vi "Parameters.vi"() -> ()   [LabVIEW 2018]
uses:
  Class 2.lvclass
panel:
  out "A/Z":dbl
  out "A/Z 3":dbl
  in  "Z2 6":dbl=3.0
  in  "A2 6":dbl=16.0
  out "Im 8":dbl format="%#.3f"
  out "B0(T) 8":dbl format="%#.3f"
  out "B0(kGs) 8":dbl format="%#.3f"
  out "MeV/u 8":dbl format="%#.3f"
  out "F 8":dbl format="%#.3f"
  out "A/Z 8":dbl format="%#.3f"
  out "E (MeV)2 6":dbl format="%#.3f"
  out "Udef 8":dbl format="%#.3f"
  out "Uinfl 8":dbl format="%#.3f"
  out "Ubender 8":dbl format="%#.3f"
  out "UIAT 8":dbl format="%#.3f"
  out "Uinj 8":dbl format="%#.3f"
  in  "Z2 5":dbl=2.0
  in  "A2 5":dbl=12.0
  out "Im 7":dbl format="%#.3f"
  out "B0(T) 7":dbl format="%#.3f"
  out "B0(kGs) 7":dbl format="%#.3f"
  out "MeV/u 7":dbl format="%#.3f"
  out "F 7":dbl format="%#.3f"
  out "A/Z 7":dbl format="%#.3f"
  out "E (MeV)2 5":dbl format="%#.3f"
  out "Udef 7":dbl format="%#.3f"
  out "Uinfl 7":dbl format="%#.3f"
  out "Ubender 7":dbl format="%#.3f"
  out "UIAT 7":dbl format="%#.3f"
  out "Uinj 7":dbl format="%#.3f"
  in  "Z":dbl=3.0
  in  "A":dbl=14.0
  out "Im 6":dbl format="%#.3f"
  out "B0(T) 6":dbl format="%#.3f"
  out "B0(kGs) 6":dbl format="%#.3f"
  out "MeV/u 6":dbl format="%#.3f"
  out "F 6":dbl format="%#.3f"
  out "A/Z 6":dbl format="%#.3f"
  out "E (MeV)2 4":dbl format="%#.3f"
  out "Udef 6":dbl format="%#.3f"
  out "Uinfl 6":dbl format="%#.3f"
  out "Ubender 6":dbl format="%#.3f"
  out "UIAT 6":dbl format="%#.3f"
  out "Uinj 6":dbl format="%#.3f"
  in  "Z2 3":dbl=3.0
  in  "A2 3":dbl=16.0
  out "Im 5":dbl format="%#.3f"
  out "B0(T) 5":dbl format="%#.3f"
  out "B0(kGs) 5":dbl format="%.3f"
  out "MeV/u 5":dbl format="%#.3f"
  out "F 5":dbl format="%#.3f"
  out "A/Z 5":dbl format="%#.3f"
  out "E (MeV)2 3":dbl format="%#.3f"
  out "Udef 5":dbl format="%#.3f"
  out "Uinfl 5":dbl format="%#.3f"
  out "Ubender 5":dbl format="%#.3f"
  out "UIAT 5":dbl format="%#.3f"
  out "Uinj 5":dbl format="%#.3f"
  out "E (MeV)2 2":dbl format="%#.3f"
  in  "Z2 2":dbl=2.0
  in  "A2 2":dbl=12.0
  out "Udef 4":dbl format="%#.3f"
  out "Uinfl 4":dbl format="%#.3f"
  out "Ubender 4":dbl format="%#.3f"
  out "UIAT 4":dbl format="%#.3f"
  out "Uinj 4":dbl format="%#.3f"
  out "Im 4":dbl format="%#.3f"
  out "B0(T) 4":dbl format="%#.3f"
  out "B0(kGs) 4":dbl format="%.3f"
  out "MeV/u 4":dbl format="%#.3f"
  out "F 4":dbl format="%#.3f"
  out "A/Z 4":dbl format="%#.3f"
  out "E (MeV)2":dbl format="%#.3f"
  in  "Z":dbl=3.0
  in  "A":dbl=14.0
  out "Udef 3":dbl format="%#.3f"
  out "Uinfl 3":dbl format="%#.3f"
  out "Ubender 3":dbl format="%#.3f"
  out "UIAT 3":dbl format="%#.3f"
  out "Uinj 3":dbl format="%#.3f"
  out "Im 3":dbl format="%#.3f"
  out "B0(T) 3":dbl format="%#.3f"
  out "B0(kGs) 3":dbl format="%.3f"
  out "MeV/u 3":dbl format="%#.3f"
  out "F 3":dbl format="%#.3f"
  in  "Rm":dbl=9.2
  out "Udef":dbl format="%#.3f"
  out "Uinfl":dbl format="%#.3f"
  out "Ubender":dbl format="%#.3f"
  out "UIAT":dbl format="%#.3f"
  out "Uinj":dbl format="%#.3f"
  out "Im":dbl format="%#.3f"
  out "B0(T)":dbl format="%#.3f"
  out "B0(kGs)":dbl format="%#.3f"
  out "MeV/u":dbl format="%#.3f"
  out "F":dbl format="%#.3f"
  out "A/Z":dbl format="%#.3f"
  in  "Rm":dbl=7.5
  out "Udef":dbl format="%#.3f"
  out "Uinfl":dbl format="%#.3f"
  out "Ubender":dbl format="%#.3f"
  out "UIAT":dbl format="%#.3f"
  out "Uinj":dbl format="%#.3f"
  out "Im":dbl format="%#.3f"
  out "B0(T)":dbl format="%#.3f"
  out "B0(kGs)":dbl format="%.3f"
  out "MeV/u":dbl format="%#.3f"
  out "F":dbl format="%#.3f"
  in  "stop":bool
  in  "HARM":dbl=3.0
  in  "UECR":dbl=15.0
  in  "E (MeV)":dbl=255.0
  in  "Rextr":dbl=1.78
  in  "Z":dbl=10.0
  in  "A":dbl=48.0
  # "Инфлектор типа A"
  # "Инфлектор типа B"
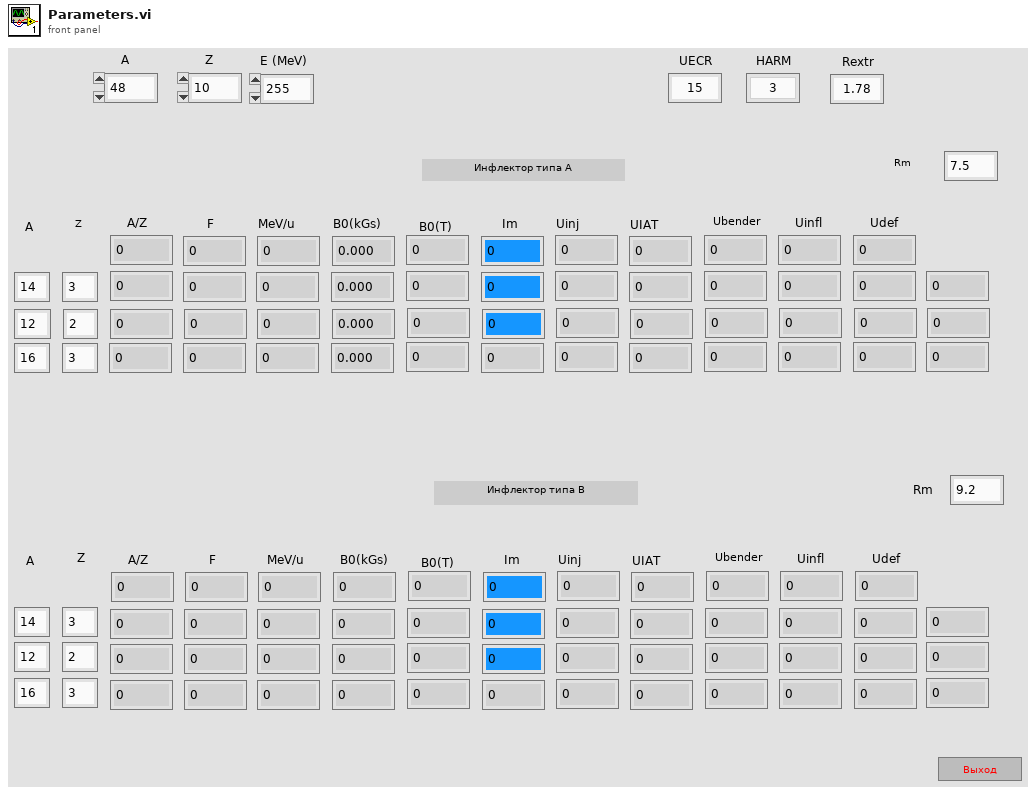
[diagram p1: front panel]
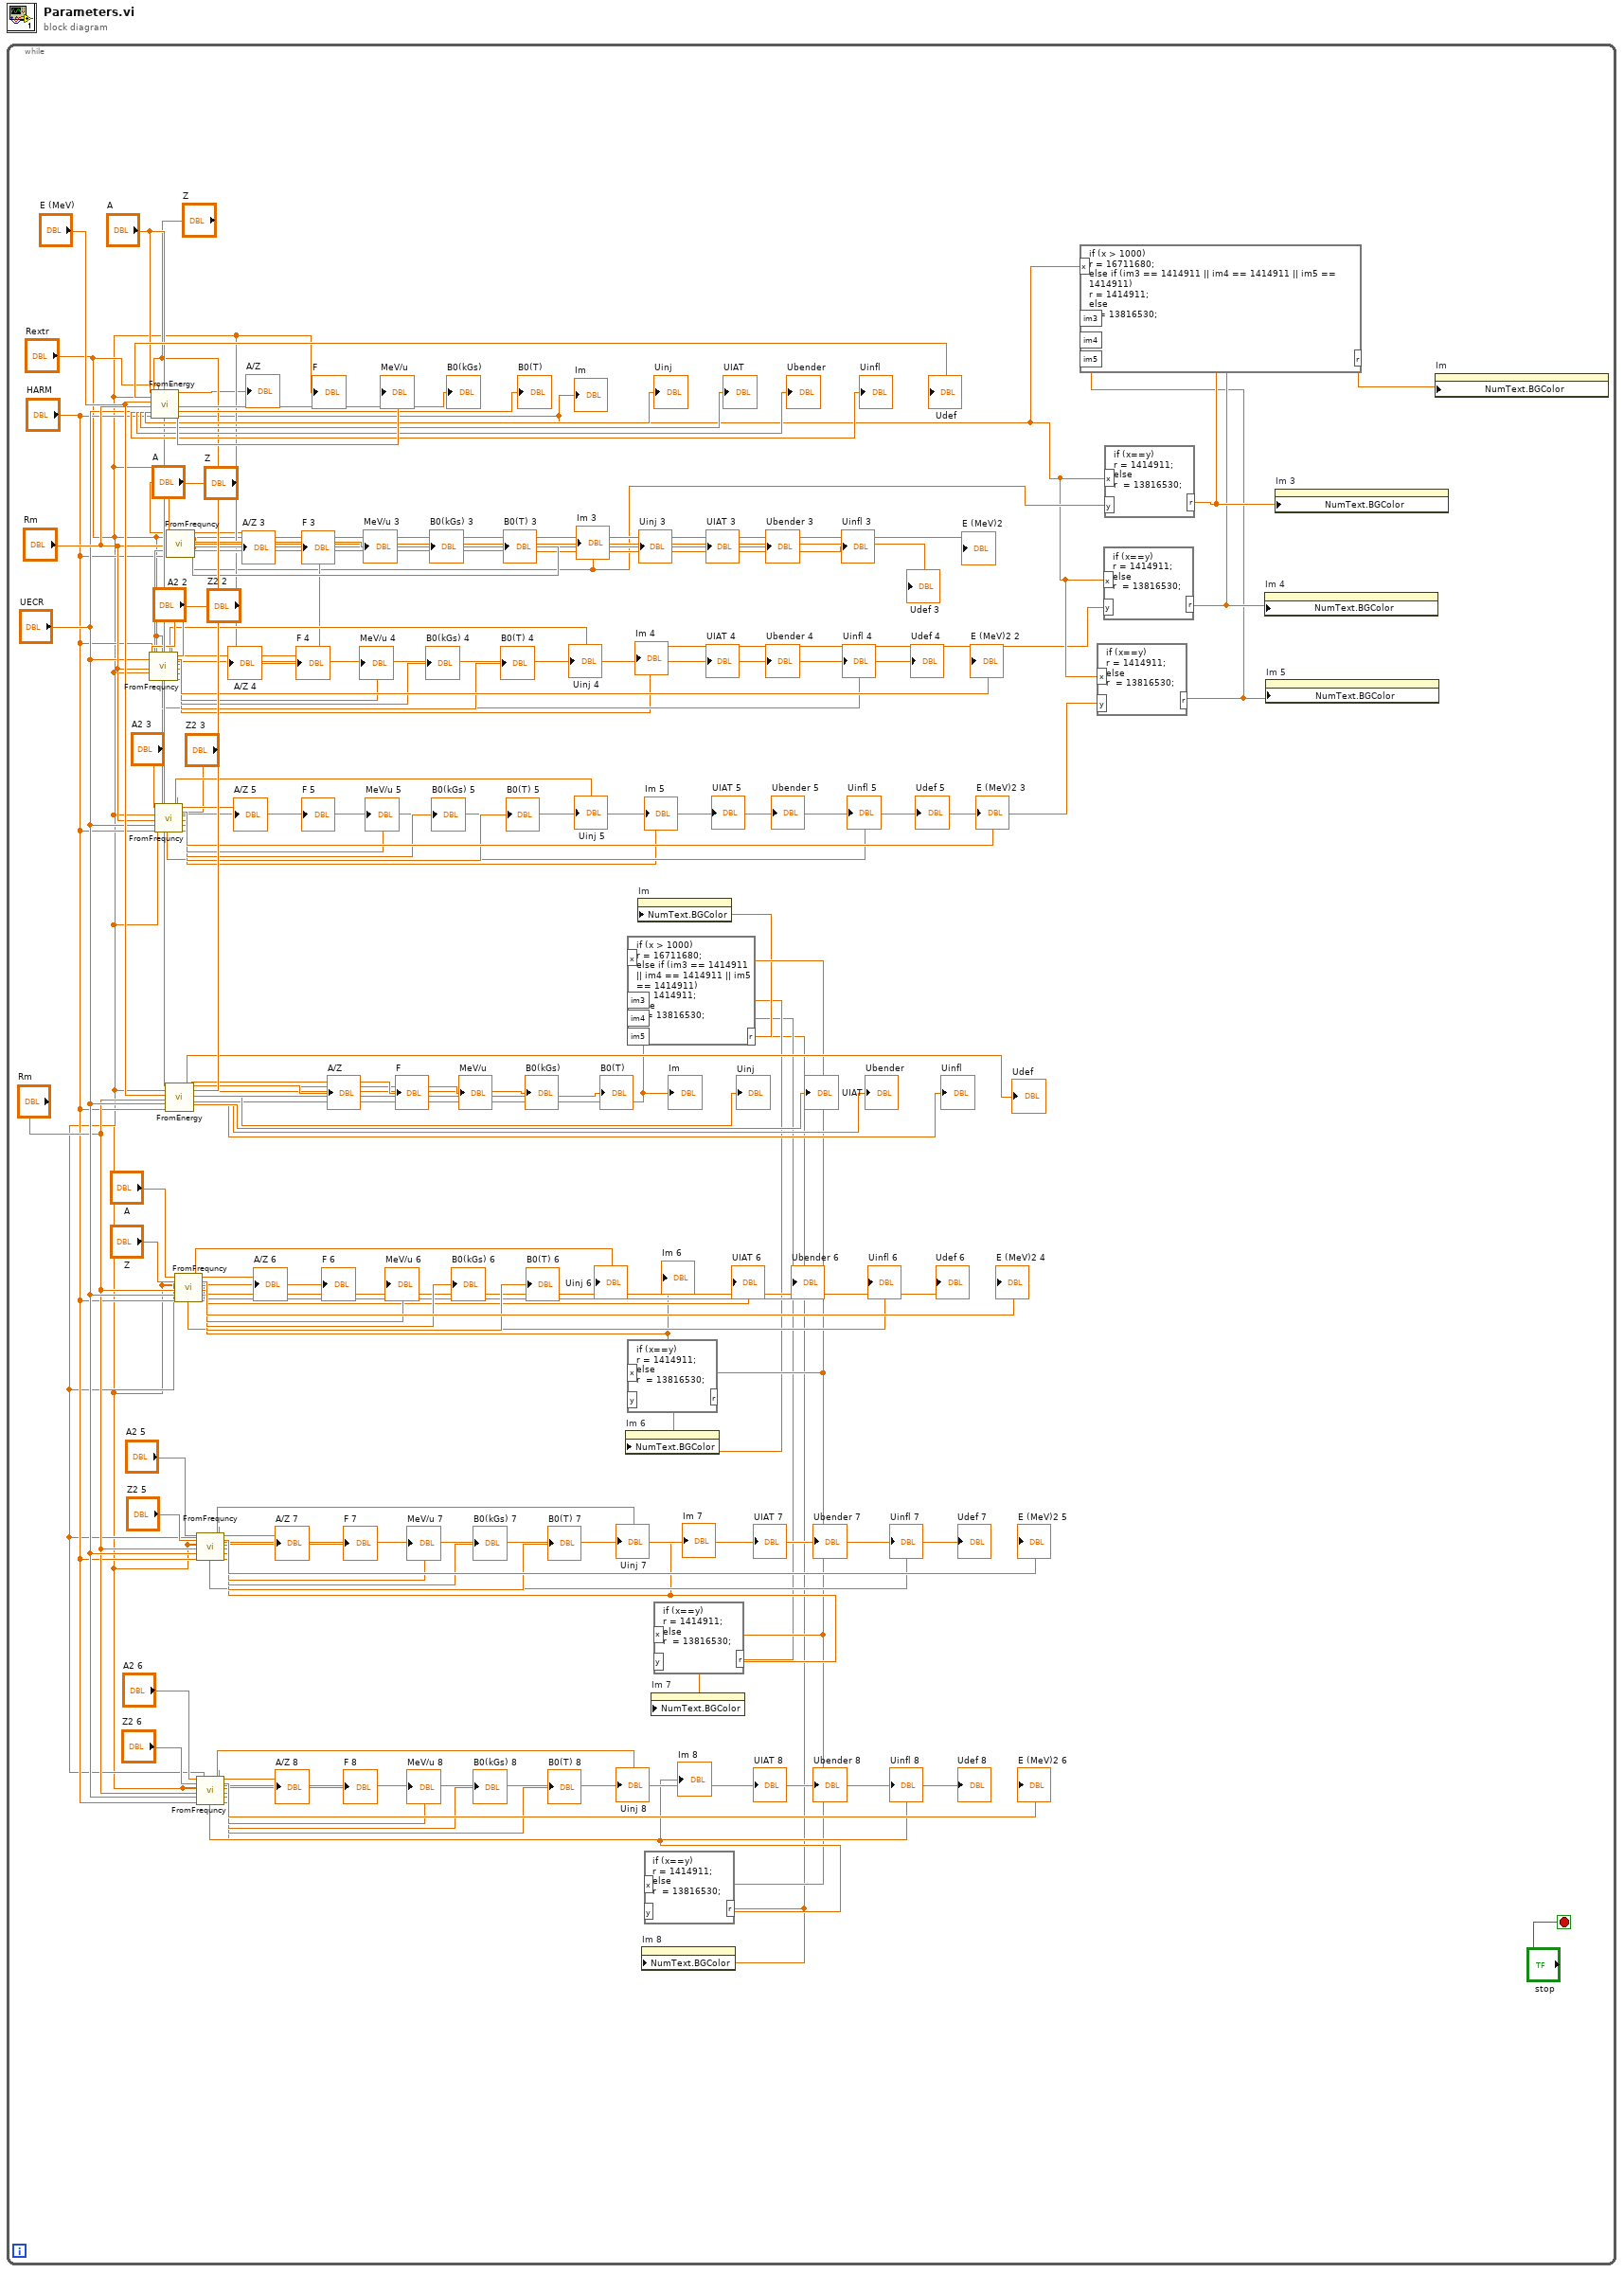
[diagram p0: block diagram]
diagram:
  n1 = while {
    stop <- "stop" stop-if-true
    n2 = call "FromEnergy.vi"("A"="A", "Z"="Z", "E (MeV)"="E (MeV)", "Rm"="Rm", "UECR"="UECR", "HARM"="HARM", "Rextr"="Rextr") -> ("Uinfl"=→"Uinfl":dbl, "Ubender"=→"Ubender":dbl, "UIAT"=→"UIAT":dbl, "Udef"=→"Udef":dbl, "Uinj"=→"Uinj":dbl, "A/Z"=→"A/Z":dbl, "F"=w20:dbl, "MeV/u"=→"MeV/u":dbl, "B0(kGs)"=→"B0(kGs)":dbl, "B0(T)"=→"B0(T)":dbl, "Im"=w14:dbl)  [unwired: 2 in]
    "F" <- w20
    "Im" <- w14
    "F 3" <- w20
    "F 4" <- w20
    "F 5" <- w20
    "F 6" <- w20
    "F 7" <- w20
    "F 8" <- w20
    n3 = call "FromFrequncy.vi"("A"="A2 2", "Z"="Z2 2", "F"=w20, "Rm"="Rm", "UECR"="UECR", "HARM"="HARM", "Rextr"="Rextr") -> ("Uinfl"=→"Uinfl 4":dbl, "Ubender"=→"Ubender 4":dbl, "UIAT"=→"UIAT 4":dbl, "Udef"=→"Udef 4":dbl, "Uinj"=→"Uinj 4":dbl, "A/Z"=→"A/Z 4":dbl, "E (MeV)"=→"E (MeV)2 2":dbl, "MeV/u"=→"MeV/u 4":dbl, "B0(kGs)"=→"B0(kGs) 4":dbl, "B0(T)"=→"B0(T) 4":dbl, "Im"=w13:dbl)  [unwired: 2 in]
    "Im 4" <- w13
    n4 = call "FromFrequncy.vi"("A"="A2 3", "Z"="Z2 3", "F"=w20, "Rm"="Rm", "UECR"="UECR", "HARM"="HARM", "Rextr"="Rextr") -> ("Uinfl"=→"Uinfl 5":dbl, "Ubender"=→"Ubender 5":dbl, "UIAT"=→"UIAT 5":dbl, "Udef"=→"Udef 5":dbl, "Uinj"=→"Uinj 5":dbl, "A/Z"=→"A/Z 5":dbl, "E (MeV)"=→"E (MeV)2 3":dbl, "MeV/u"=→"MeV/u 5":dbl, "B0(kGs)"=→"B0(kGs) 5":dbl, "B0(T)"=→"B0(T) 5":dbl, "Im"=w12:dbl)  [unwired: 2 in]
    "Im 5" <- w12
    n5 = call "FromEnergy.vi"("A"="A", "Z"="Z", "E (MeV)"="E (MeV)", "Rm"="Rm", "UECR"="UECR", "HARM"="HARM", "Rextr"="Rextr") -> ("Uinfl"=→"Uinfl":dbl, "Ubender"=→"Ubender":dbl, "UIAT"=→"UIAT":dbl, "Udef"=→"Udef":dbl, "Uinj"=→"Uinj":dbl, "A/Z"=→"A/Z":dbl, "F"=→"F":dbl, "MeV/u"=→"MeV/u":dbl, "B0(kGs)"=→"B0(kGs)":dbl, "B0(T)"=→"B0(T)":dbl, "Im"=w5:dbl)  [unwired: 2 in]
    "Im" <- w5
    n6 = call "FromFrequncy.vi"("A"="A", "Z"="Z", "F"=w20, "Rm"="Rm", "UECR"="UECR", "HARM"="HARM", "Rextr"="Rextr") -> ("Uinfl"=→"Uinfl 3":dbl, "Ubender"=→"Ubender 3":dbl, "UIAT"=→"UIAT 3":dbl, "Udef"=→"Udef 3":dbl, "Uinj"=→"Uinj 3":dbl, "A/Z"=→"A/Z 3":dbl, "E (MeV)"=→"E (MeV)2":dbl, "MeV/u"=→"MeV/u 3":dbl, "B0(kGs)"=→"B0(kGs) 3":dbl, "B0(T)"=→"B0(T) 3":dbl, "Im"=w16:dbl)  [unwired: 2 in]
    "Im 3" <- w16
    n7 = call "FromFrequncy.vi"("A"="A", "Z"="Z", "F"=w20, "Rm"="Rm", "UECR"="UECR", "HARM"="HARM", "Rextr"="Rextr") -> ("Uinfl"=→"Uinfl 6":dbl, "Ubender"=→"Ubender 6":dbl, "UIAT"=→"UIAT 6":dbl, "Udef"=→"Udef 6":dbl, "Uinj"=→"Uinj 6":dbl, "A/Z"=→"A/Z 6":dbl, "E (MeV)"=→"E (MeV)2 4":dbl, "MeV/u"=→"MeV/u 6":dbl, "B0(kGs)"=→"B0(kGs) 6":dbl, "B0(T)"=→"B0(T) 6":dbl, "Im"=w8:dbl)  [unwired: 2 in]
    "Im 6" <- w8
    n8 = call "FromFrequncy.vi"("A"="A2 5", "Z"="Z2 5", "F"=w20, "Rm"="Rm", "UECR"="UECR", "HARM"="HARM", "Rextr"="Rextr") -> ("Uinfl"=→"Uinfl 7":dbl, "Ubender"=→"Ubender 7":dbl, "UIAT"=→"UIAT 7":dbl, "Udef"=→"Udef 7":dbl, "Uinj"=→"Uinj 7":dbl, "A/Z"=→"A/Z 7":dbl, "E (MeV)"=→"E (MeV)2 5":dbl, "MeV/u"=→"MeV/u 7":dbl, "B0(kGs)"=→"B0(kGs) 7":dbl, "B0(T)"=→"B0(T) 7":dbl, "Im"=w7:dbl)  [unwired: 2 in]
    "Im 7" <- w7
    n9 = call "FromFrequncy.vi"("A"="A2 6", "Z"="Z2 6", "F"=w20, "Rm"="Rm", "UECR"="UECR", "HARM"="HARM", "Rextr"="Rextr") -> ("Uinfl"=→"Uinfl 8":dbl, "Ubender"=→"Ubender 8":dbl, "UIAT"=→"UIAT 8":dbl, "Udef"=→"Udef 8":dbl, "Uinj"=→"Uinj 8":dbl, "A/Z"=→"A/Z 8":dbl, "E (MeV)"=→"E (MeV)2 6":dbl, "MeV/u"=→"MeV/u 8":dbl, "B0(kGs)"=→"B0(kGs) 8":dbl, "B0(T)"=→"B0(T) 8":dbl, "Im"=w6:dbl)  [unwired: 2 in]
    "Im 8" <- w6
    n10 = formula code="if (x==y)\nr = 1414911;\nelse\nr  = 13816530;"("x"=w5, "y"=w8) -> ("r"=w3:dbl)
    n11 = property on="Im 6" class="DigNum (strict)"("NumText.BGColor"=w3) -> ()  [unwired: 2 in, 2 out]
    n12 = formula code="if (x==y)\nr = 1414911;\nelse\nr  = 13816530;"("x"=w5, "y"=w6) -> ("r"=w1:dbl)
    n13 = property on="Im 8" class="DigNum (strict)"("NumText.BGColor"=w1) -> ()  [unwired: 2 in, 2 out]
    n14 = formula code="if (x==y)\nr = 1414911;\nelse\nr  = 13816530;"("x"=w5, "y"=w7) -> ("r"=w2:dbl)
    n15 = formula code="if (x > 1000)\nr = 16711680;\nelse if (im3 == 1414911 || im4 == 1414911 || im5 == 1414911)\nr = 1414911;\nelse\nr  = 13816530;"("x"=w5, "im3"=w3, "im4"=w2, "im5"=w1) -> ("r"=w4:dbl)
    n16 = property on="Im" class="DigNum (strict)"("NumText.BGColor"=w4) -> ()  [unwired: 2 in, 2 out]
    n17 = property on="Im 7" class="DigNum (strict)"("NumText.BGColor"=w2) -> ()  [unwired: 2 in, 2 out]
    n18 = formula code="if (x==y)\nr = 1414911;\nelse\nr  = 13816530;"("x"=w14, "y"=w12) -> ("r"=w9:dbl)
    n19 = formula code="if (x==y)\nr = 1414911;\nelse\nr  = 13816530;"("x"=w14, "y"=w13) -> ("r"=w10:dbl)
    n20 = formula code="if (x==y)\nr = 1414911;\nelse\nr  = 13816530;"("x"=w14, "y"=w16) -> ("r"=w11:dbl)
    n21 = formula code="if (x > 1000)\nr = 16711680;\nelse if (im3 == 1414911 || im4 == 1414911 || im5 == 1414911)\nr = 1414911;\nelse\nr  = 13816530;"("x"=w14, "im3"=w11, "im4"=w10, "im5"=w9) -> ("r"=w15:dbl)
    n22 = property on="Im 4" class="Digital (strict)"("NumText.BGColor"=w10) -> ()  [unwired: 2 in, 2 out]
    n23 = property on="Im 5" class="Digital (strict)"("NumText.BGColor"=w9) -> ()  [unwired: 2 in, 2 out]
    n24 = property on="Im 3" class="Digital (strict)"("NumText.BGColor"=w11) -> ()  [unwired: 2 in, 2 out]
    n25 = property on="Im" class="Digital (strict)"("NumText.BGColor"=w15) -> ()  [unwired: 2 in, 2 out]
  }
